vi "S8300E_RawFiles2_txt.vi"() -> ()   [LabVIEW 2011]
uses:
  Instance           1 30Saved   KT300WR2_RawFiles2_txt .vi
panel:
  out "Prefix_FileName":string
  out "Total txt  Files":i32
  out "Status":string
  out "txt File List":string[](array[string])
  out "file names":string[](array[string])
  out "size(s)":i32
  out "spreadsheet string":string
  out "Title Form":string
  out "String":string
  out "appended array":T1(array[cluster])
  out "Remove String":string
  out "output string":string
  out "PickLineNo":i32
  out "Search String":string="USN="
  out "Data":string
  out "text":string
  out "Begin time":u32
  # "S8300E  Raw Files to a Txt File"
  # "2015-4-8"
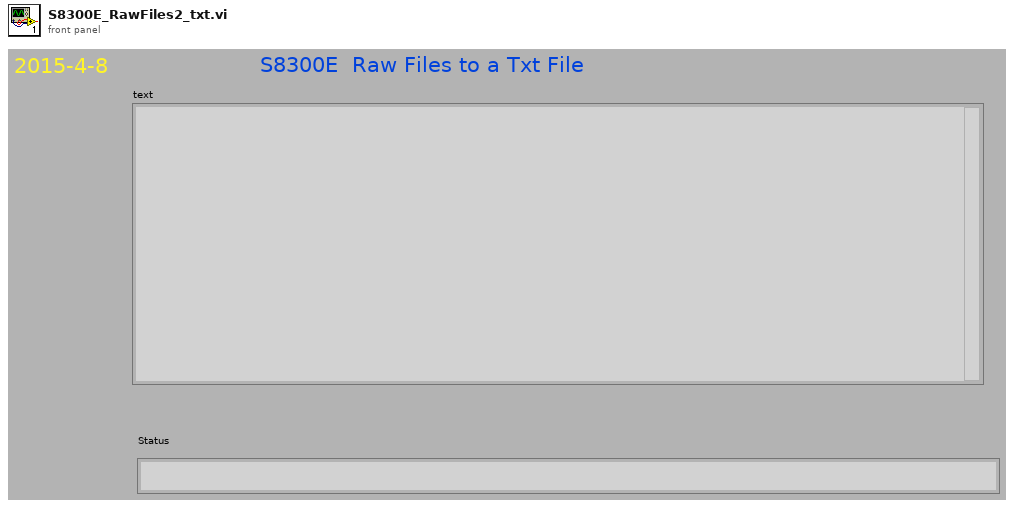
[diagram p1: front panel]
types:
  T1 = cluster{string, i32, "regular expression (\"\")":string}[]
  T2 = enum32{"invalid app kind", "Development System", "Run Time System", "Student Edition", "Embedded LabVIEW", "Evaluation", "Custom"}
  T3 = cluster{string, i32, "regular expression (\"\")":string}
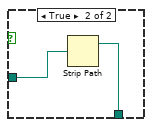
[diagram p3: hidden frame]
diagram:
  (unwired) "TP75  Voltage=4.944103\nTP73  Voltage=9.060578\nTP74  Voltage=4.949983\nTP76  Voltage=3.343905\nTP78  Voltage=1.289406\nTP72  Voltage=6.938396"
  n1 = flat-sequence {
    tunnel: [w192] -> w1
    tunnel: w1 -> [w234]
    frame #0 {
      n2 = Tick Count (ms)() -> (millisecond timer value=→"Begin time":u32)
      "Status" <- ""
    }
    frame #1 {
      n3 = call "Prompt User for Input"() -> ("Prefix_FileName"=→"Prefix_FileName":string)  [unwired: 17 in, 2 out]
    }
    frame #2 {
      n4 = Current VI's Path() -> (path=w17:path)
      n5 = Strip Path(path=w17) -> (stripped path=w13:path)  [unwired: 1 out]
      n6 = property class="App"() -> ("App.Kind"=w14:T2)  [unwired: 2 in, 2 out]
      n7 = Equal?(x=w14, y=T2."Run Time System" ("Application:Kind")) -> (x = y?=w16:bool)
      n8 = case shown="False" w16 {
        tunnel: [w39 w41] -> w12
        tunnel: w13 -> [w39 w40]
        frame False {
        }
        frame True {
          n9 = Strip Path(path=w40) -> (stripped path=w41:path)  [unwired: 1 out]
        }
      }
      n10 = List Folder(path=w12) -> (filenames=w6:string[])  [unwired: 3 in, 3 out]
      "file names" <- w6
      n11 = Concatenate Strings("%s" ("format string"), "\n") -> (w9:string)
      n12 = Array To Spreadsheet String(array=w6, 3:w9) -> (spreadsheet string=→"spreadsheet string":string)  [unwired: 1 in]
      n13 = Array Size(array=w6) -> (size(s)=w7:i32)
      "size(s)" <- w7
      n14 = for {
        N: w7 -> [_]
        shift-right: [w19] -> _
        shift-left: string[] [] -> [w20]
        i -> [w35]
        n15 = local read "file names"() -> (w34:string[])
        n16 = local read "Prefix_FileName"() -> (w18:string)
        n17 = Index Array(array=w34, index=w35) -> (element=w21:string)
        n18 = call <vilib>:"Trim Whitespace.vi"("string"=".txt") -> ("trimmed string"=w28:string)  [unwired: 1 in]
        n19 = call <vilib>:"Trim Whitespace.vi"("string"=w18) -> ("trimmed string"=w32:string)  [unwired: 1 in]
        n20 = call <vilib>:"Trim Whitespace.vi"("string"=w21) -> ("trimmed string"=w33:string)  [unwired: 1 in]
        n21 = To Upper Case(1:w28) -> (0:w25:string)
        n22 = To Upper Case(1:w32) -> (0:w30:string)
        n23 = To Upper Case(1:w33) -> (0:w29:string)
        n24 = Match Pattern(string=w29, regular expression=w30) -> (match substring=w31:string)  [unwired: 1 in, 3 out]
        n25 = Match Pattern(string=w29, regular expression=w25) -> (match substring=w26:string)  [unwired: 1 in, 3 out]
        n26 = Equal?(x=w31, y=w30) -> (x = y?=w24:bool)
        n27 = Equal?(x=w26, y=w25) -> (x = y?=w23:bool)
        n28 = And(x=w24, y=w23) -> (x .and. y?=w22:bool)
        n29 = case shown="True" w22 {
          tunnel: w21 -> [_ w38]
          tunnel: w20 -> [_ w36]
          tunnel: [_ w37] -> w19
          frame False {
          }
          frame True {
            n30 = Build Array (concatenate) "Build Array"(w36, w38) -> (w37:string[])
            "txt File List" <- w37
          }
        }
      }
    }
    frame #3 {
      n31 = local read "txt File List"() -> (w44:string[])
      n32 = Array Size(array=w44) -> (size(s)=w43:i32)
      "Total txt  Files" <- w43
      n33 = Equal To 0?(x=w43) -> (x = 0?=w42:bool)
      n34 = case shown="True" w42 {
        frame False {
        }
        frame True {
          n35 = flat-sequence {
            frame #0 {
              n36 = call "Display Message to User"() -> ()  [unwired: 10 in, 2 out]
            }
            frame #1 {
              n37 = Stop(stop? (T)=TRUE) -> ()
            }
          }
        }
      }
    }
    frame #4 {
      w135 = ""
      w138 = 0
      w139 = "USN="
      n38 = Bundle("P3V3_PCH=", 0, "") -> (w59:cluster{string, i32, string})  [unwired: 1 in]
      n39 = Bundle("P1V8_PCH=", 0, "") -> (w60:cluster{string, i32, string})  [unwired: 1 in]
      n40 = Bundle("H-P1V5=", 0, "") -> (w58:cluster{string, i32, string})  [unwired: 1 in]
      n41 = Bundle("MB Temp=", 0, "") -> (w46:cluster{string, i32, string})  [unwired: 1 in]
      n42 = Bundle("DDR3-2T Temp=", 0, "") -> (w47:cluster{string, i32, string})  [unwired: 1 in]
      n43 = Bundle("DDR3-1T Temp=", 0, "") -> (w48:cluster{string, i32, string})  [unwired: 1 in]
      n44 = Bundle("L-P1V5=", 0, "") -> (w105:cluster{string, i32, string})  [unwired: 1 in]
      n45 = Bundle("PVCCSA=", 0, "") -> (w106:cluster{string, i32, string})  [unwired: 1 in]
      n46 = Bundle("L-P0V75=", 0, "") -> (w104:cluster{string, i32, string})  [unwired: 1 in]
      n47 = Bundle("P1V8=", 0, "") -> (w109:cluster{string, i32, string})  [unwired: 1 in]
      n48 = Bundle("P1V0_PCH=", 0, "") -> (w107:cluster{string, i32, string})  [unwired: 1 in]
      n49 = Bundle("PVCCPLL=", 0, "") -> (w102:cluster{string, i32, string})  [unwired: 1 in]
      n50 = Bundle("PVCCIO=", 0, "") -> (w108:cluster{string, i32, string})  [unwired: 1 in]
      n51 = Bundle("P5V=", 0, "") -> (w131:cluster{string, i32, string})  [unwired: 1 in]
      n52 = Bundle("P3V3=", 0, "") -> (w110:cluster{string, i32, string})  [unwired: 1 in]
      n53 = Bundle("H-P0V75=", 0, "") -> (w82:cluster{string, i32, string})  [unwired: 1 in]
      n54 = Bundle("CPU1 Temp=", 0, "") -> (w81:cluster{string, i32, string})  [unwired: 1 in]
      n55 = Bundle(w139, w138, w135) -> (w132:cluster{string, i32, string})  [unwired: 1 in]
      n56 = Bundle("P1V5_PCH=", 0, "") -> (w83:cluster{string, i32, string})  [unwired: 1 in]
      n57 = Bundle("CPU2 Temp=", 0, "") -> (w80:cluster{string, i32, string})  [unwired: 1 in]
      n58 = Bundle("PCH  Temp=", 0, "") -> (w79:cluster{string, i32, string})  [unwired: 1 in]
      n59 = Bundle("P3V3_S0=", 0, "") -> (w85:cluster{string, i32, string})  [unwired: 1 in]
      n60 = Bundle("P1V05_PCH=", 0, "") -> (w84:cluster{string, i32, string})  [unwired: 1 in]
      n61 = Build Array "Build Array"(w132, w131, w110, w109, w108, w107, w106, w105, w104, w102, w85, w84, w83, w60, w59, w58, w82, w81, w80, w79, w48, w47, w46) -> (→"appended array":cluster{string, i32, string}[])
      n62 = local write "Title Form"("") -> ()
      "Search String" <- w139
      "PickLineNo" <- w138
      "Remove String" <- w135
    }
    frame #5 {
      w144 = "\t"
      n63 = Concatenate Strings("DDR3 SLOT2 TEMP(c)", w144) -> (w142:string)
      n64 = Concatenate Strings("DDR3 SLOT1 TEMP(c)", w144) -> (w143:string)
      n65 = Concatenate Strings("MB TEMP(c)", w144) -> (w141:string)
      n66 = Concatenate Strings("P3V3_PCH", w144) -> (w148:string)
      n67 = Concatenate Strings("P1V8_PCH", w144) -> (w149:string)
      n68 = Concatenate Strings("DUT_SN" ("string"), "\t") -> (w170:string)
      n69 = Concatenate Strings("PVCCIO", w144) -> (w166:string)
      n70 = Concatenate Strings("L-P1V5", w144) -> (w163:string)
      n71 = Concatenate Strings("P1V8", w144) -> (w167:string)
      n72 = Concatenate Strings("L-P0V75", w144) -> (w162:string)
      n73 = Concatenate Strings("PVCCSA", w144) -> (w164:string)
      n74 = Concatenate Strings("P3V3", w144) -> (w168:string)
      n75 = Concatenate Strings("P1V0_PCH", w144) -> (w165:string)
      n76 = Concatenate Strings("P5V", w144) -> (w169:string)
      n77 = Concatenate Strings("P1V5_PCH", w144) -> (w158:string)
      n78 = Concatenate Strings("H-P0V75", w144) -> (w157:string)
      n79 = Concatenate Strings("H-P1V5", w144) -> (w151:string)
      n80 = Concatenate Strings("P3V3_S0", w144) -> (w160:string)
      n81 = Concatenate Strings("P1V05_PCH", w144) -> (w159:string)
      n82 = Concatenate Strings("CPU2 TEMP(c)", w144) -> (w155:string)
      n83 = Concatenate Strings("CPU1 TEMP(c)", w144) -> (w156:string)
      n84 = Concatenate Strings("PVCCPLL", w144) -> (w161:string)
      n85 = Concatenate Strings("PCH  TEMP(c)", w144) -> (w154:string)
      n86 = Concatenate Strings(w170, w169, w168, w167, w166, w165, w164, w163, w162, w161, w160, w159, w158, w149, w148, w151, w157, w156, w155, w154, w143, w142, w141, "\n") -> (→"Title Form":string)
    }
    frame #6 {
      n87 = local write "Data"("") -> ()
    }
    frame #7 {
      n88 = local read "Total txt  Files"() -> (w191:i32)
      n89 = for {
        N: w191 -> [_]
        shift-right: [w197] -> w192
        shift-left: "" -> [w195]
        i -> [w196]
        n90 = local read "appended array"() -> (w205:T1)
        n91 = local read "txt File List"() -> (w201:string[])
        n92 = Array Size(array=w205) -> (size(s)=w204:i32)
        n93 = Index Array(array=w201, index=w196) -> (element=w198:string)
        n94 = call "SUB_Read_specifFile.vi"("name or relative path"=w198) -> ("text"=w206:string)  [unwired: 1 in, 1 out]
        "text" <- w206
        n95 = for {
          N: w204 -> [_]
          tunnel: w206 -> [w227]
          tunnel: w205 -> [w222]
          shift-right: [w216] -> w202
          shift-left: "" -> [w217]
          i -> [w215]
          (unwired) TRUE ("replace all? (F)")
          n96 = Index Array(array=w222, index=w215) -> (element=w221:T3)
          n97 = Unbundle(w221) -> (w218:string, w220:i32, "regular expression (\"\")"=w219:string)
          n98 = call "SUB_FindSpecificString.vi"("Find this String"=w218, "String data"=w227) -> ("before \"; \" string"=w226:string, "Found"=w210:bool)  [unwired: 2 in]
          n99 = Pick Line(multi-line string=w226, line index=w220) -> (output string=w225:string)  [unwired: 1 in]
          "output string" <- w225
          n100 = Search and Replace String(replace all?=TRUE ("replace all? (F)"), input string=w225, search string=w219, replace string="") -> (result string=w207:string)  [unwired: 4 in, 3 out]
          "Data" <- w207
          n101 = String Length(string=w207) -> (length=w213:i32)
          n102 = Not(x=w210) -> (.not. x?=w211:bool)
          n103 = Equal To 0?(x=w213) -> (x = 0?=w212:bool)
          n104 = Or(x=w212, y=w211) -> (x .or. y?=w209:bool)
          n105 = case shown="True" w209 {
            tunnel: [w228 "   "] -> w208
            tunnel: w207 -> [w228 _]
            frame False {
            }
            frame True {
            }
          }
          n106 = Concatenate Strings(w217, w208, "\t") -> (w216:string)
        }
        n107 = Concatenate Strings("正在解析" ("string"), w198) -> (w199:string)
        n108 = local write "Status"(w199) -> ()
        n109 = Concatenate Strings "Concatenate Strings"(w195, w202, "\r") -> (w197:string)
      }
    }
    frame #8 {
      n110 = local read "Prefix_FileName"() -> (w232:string)
      n111 = local read "Title Form"() -> (w235:string)
      n112 = Concatenate Strings(w235, w234) -> (w233:string)
      "String" <- w233
      n113 = Concatenate Strings(w232, "all_TestResult.xls" ("string")) -> (w230:string)
      n114 = call "SUB_Write_GeneralFile.vi"("Filename"=w230, "Text Input"=w233) -> ()  [unwired: 1 out]
    }
    frame #9 {
      n115 = local write "Status"("完成" ("Status")) -> ()
    }
    frame #10 {
      n116 = Quit LabVIEW(quit? (T)=FALSE) -> ()
    }
  }
